vi "SUB_COM1Wrt.vi"(0 "VISA resource name":refnum<visa-resource-name>, 1 "write buffer":string) -> (2 "duplicate VISA resource name":refnum<visa-resource-name>, 4 "return count":u32)   [LabVIEW 2011]
panel:
  out "error out":errorcluster
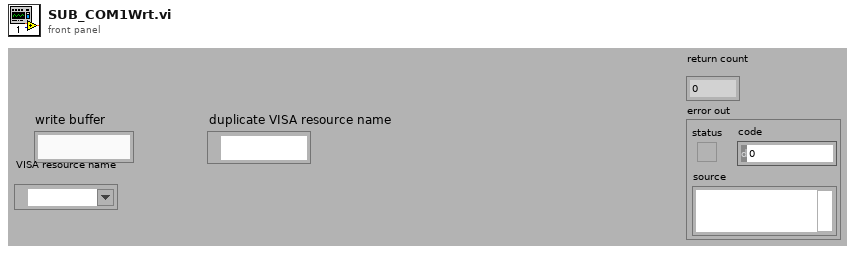
[diagram p1: front panel]
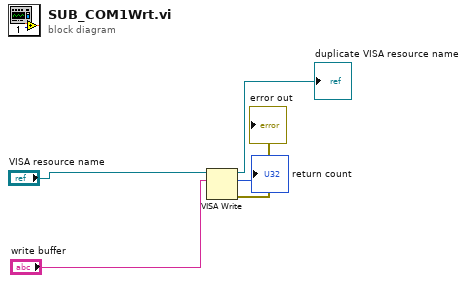
[diagram p0: block diagram]
diagram:
  n1 = VISA Write(VISA resource name="VISA resource name", write buffer="write buffer") -> (VISA resource name out=→"duplicate VISA resource name":refnum<visa-resource-name>, return count=→"return count":u32, error out=→"error out":errorcluster)  [unwired: 1 in]
